vi "Main.vi"() -> ()   [LabVIEW 2020]
doc: "This template is for the Queued Message Handler design pattern.\n\nThe Event Handling Loop generates messages based on user interface actions.\n\nThe Message Handling Loop processes messages generated by the Event Handling Loop, or by other messages. The messages are string values, so new messages can be added easily to the Message Cases case structure in the Message Handling Loop. Each message cluster can also provide an optional value for Message Data, which is a variant that can be converted to whatever message-specific data is required."
uses:
  controls/Pressure Gauge.ctl
  controls/UI Data.ctl
  controls/UI State.ctl
  Settings/Settings.ctl
  controls/Hardware Configuration.ctl
  Logging/Logging Configuration.ctl
  <vilib>/Utility/error.llb/Error Cluster From Error Code.vi
  <vilib>/ErrorRing/Error Ring.xnode
  support/Message Queue/Message Queue.lvlib
  support/User Event - Stop/User Event - Stop.lvlib
  Acquisition/Acquisition.lvlib
  Control/Control.lvlib
  Logging/Logging.lvlib
  Settings/Settings.lvlib
panel:
  out "Valve State":bool[](array[boolean])
  out "T=":dbl format="%.2g"
  in  "Run Valve Sequence":bool
  out "P X-Ducer 7":dbl(knob) scale=0.0..5000.0 scale format="%.1p"
  out "P X-Ducer 6":dbl(knob) scale=0.0..5000.0 scale format="%.1p"
  out "P X-Ducer 5":dbl(knob) scale=0.0..5000.0 scale format="%.1p"
  out "P X-Ducer 4":dbl(knob) scale=0.0..5000.0 scale format="%.1p"
  out "P X-Ducer 3":dbl(knob) scale=0.0..5000.0 scale format="%.1p"
  out "P X-Ducer 2":dbl(knob) scale=0.0..5000.0 scale format="%.1p"
  out "P X-Ducer 1":dbl(knob) scale=0.0..5000.0 scale format="%.1p"
  out "P X-Ducer 0":T1 scale=0.0..5000.0 scale format="%.1p"
  in  "Settings":bool
  in  "Start":bool
  in  "Exit":bool
  # "River City Rocketry"
  # "Liquid Propulsion System Acquisition & Control"
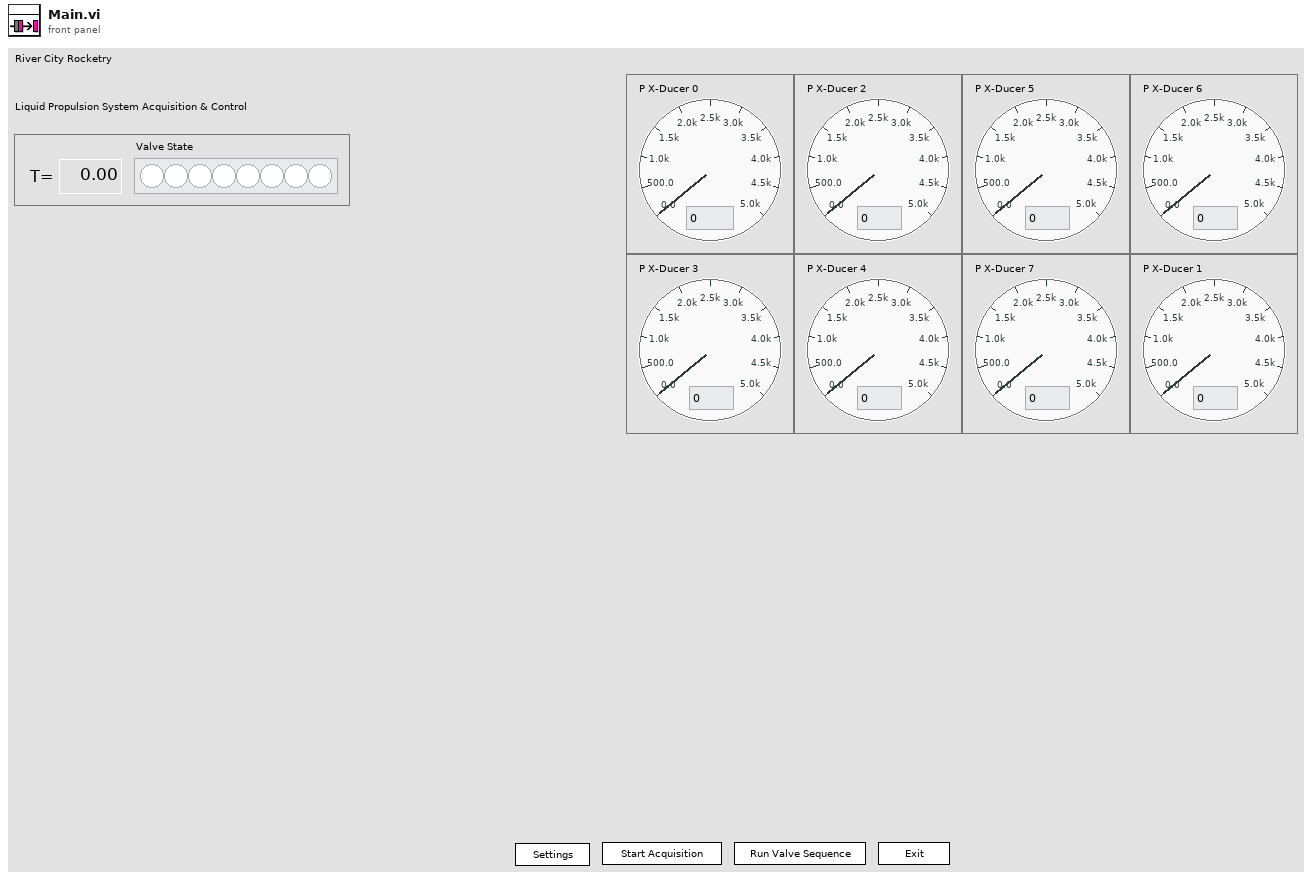
[diagram p1: front panel]
types:
  T1 = typedef "Pressure Gauge.ctl" = dbl
  T2 = typedef "Settings.lvlib/Settings.ctl" = cluster{"Hardware Configuration":T3, "Logging Configuration":T4}
  T3 = typedef "Acquisition.lvlib/Hardware Configuration.ctl" = cluster{"DAQmx Task":refnum<k21>, "Boolean":bool}
  T4 = typedef "Logging.lvlib/Logging Configuration.ctl" = cluster{"Log File Base Path":path, "TDMS File Reference":refnum<k34>, "Samples to Save":u32}
  T5 = typedef "UI State.ctl" = enum16{"Idle", "Acquiring and Logging", "Waiting for Exit", "Waiting for Exit (Acq Stopped)", "Waiting for Exit (Log Stopped)", "Waiting for Stop", "Waiting for Stop (Acq Stopped)", "Waiting for Stop (Log Stopped)"}
  T6 = typedef "UI Data.ctl" = cluster{"Settings Button Ref":refnum<vi>, "Start Button Ref":refnum<vi>, "Knob Refnum":refnum<vi>, "Knob Refnum 2":refnum<vi>, "Knob Refnum 3":refnum<vi>, "Knob Refnum 4":refnum<vi>, "Knob Refnum 5":refnum<vi>, "Knob Refnum 6":refnum<vi>, "Knob Refnum 7":refnum<vi>, "Knob Refnum 8":refnum<vi>, "Exit Button Refnum":refnum<vi>}
  T7 = typedef "Message Queue.lvlib/All Message Queues.ctl" = cluster{"Acquisition":refnum<queue>, "UI":refnum<queue>, "Control":refnum<queue>, "Logging":refnum<queue>}
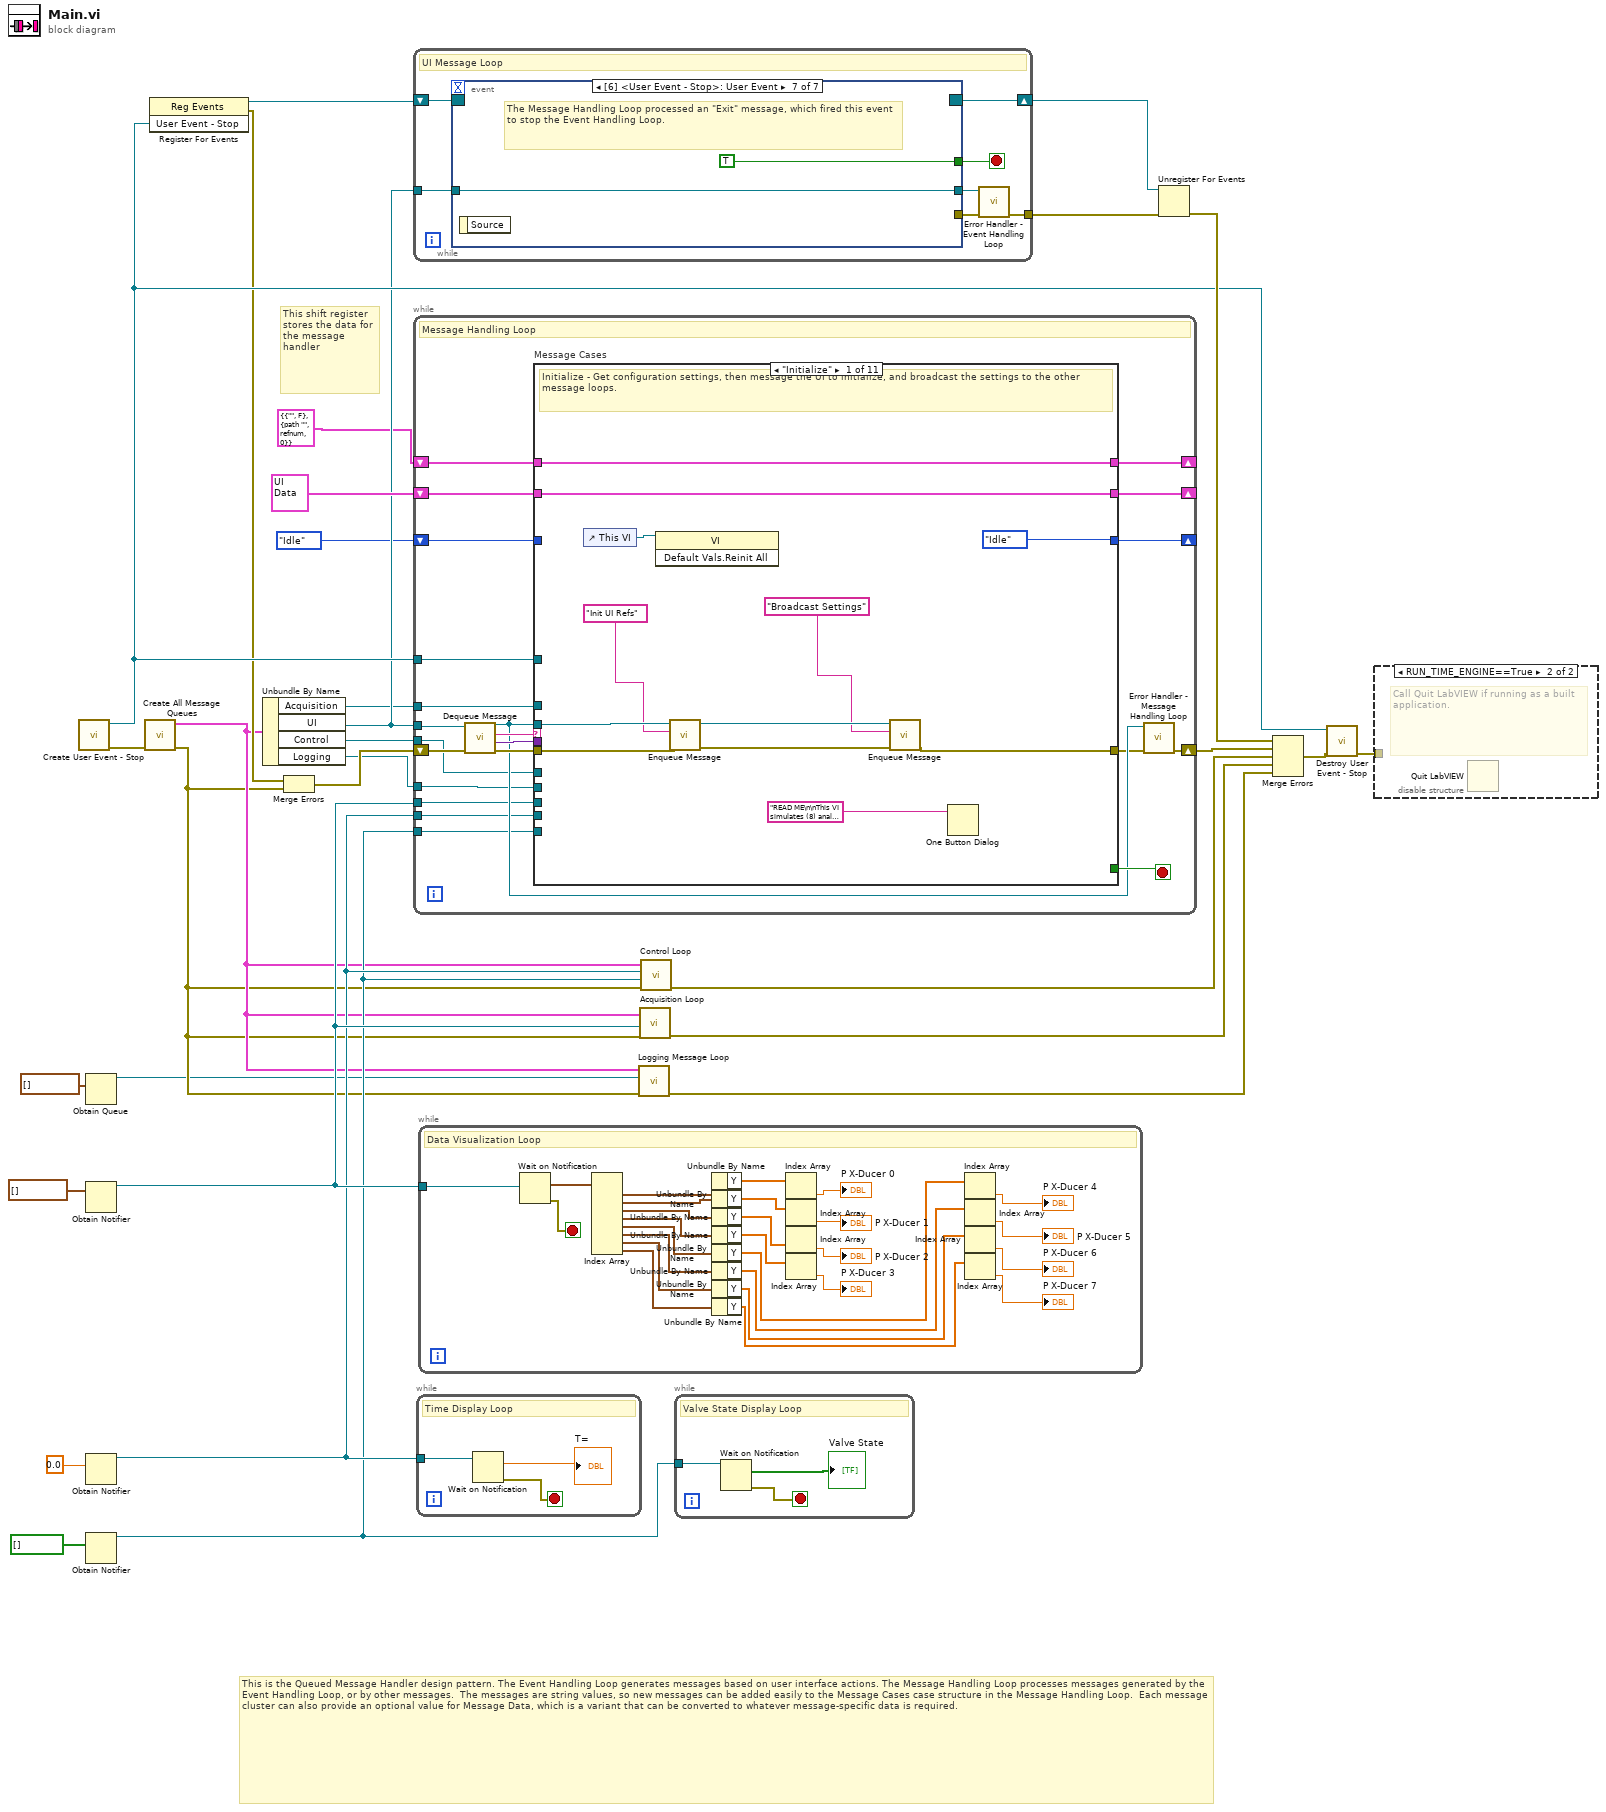
[diagram p0: block diagram]
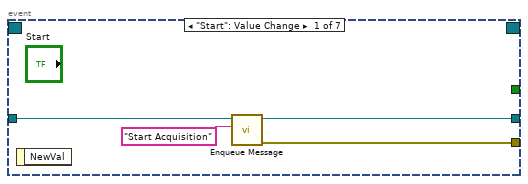
[diagram p3: hidden frame]
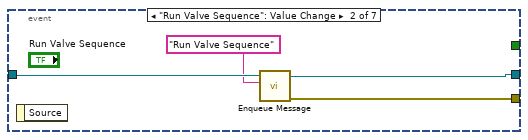
[diagram p4: hidden frame]
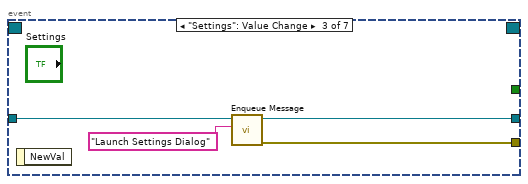
[diagram p5: hidden frame]
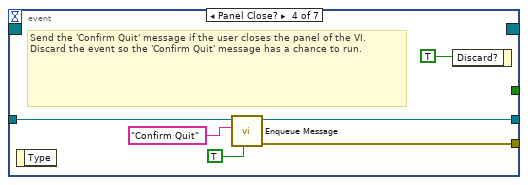
[diagram p6: hidden frame]
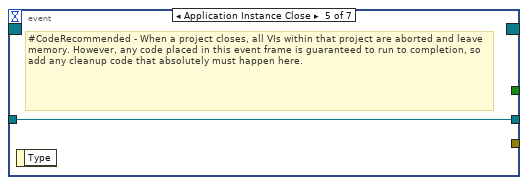
[diagram p7: hidden frame]
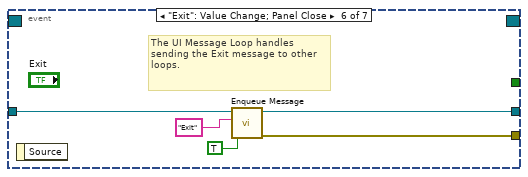
[diagram p8: hidden frame]
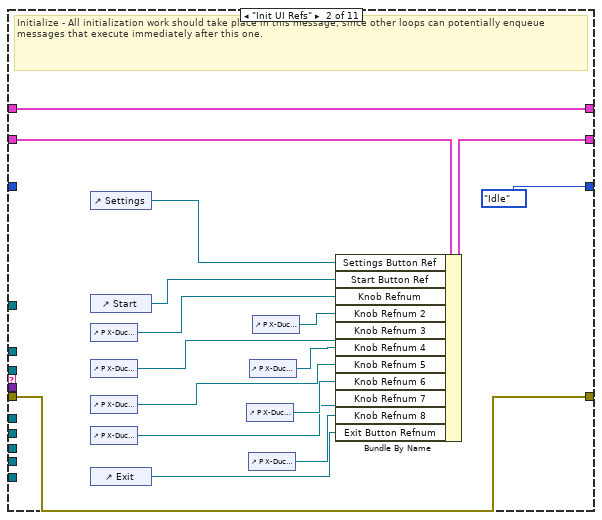
[diagram p9: hidden frame]
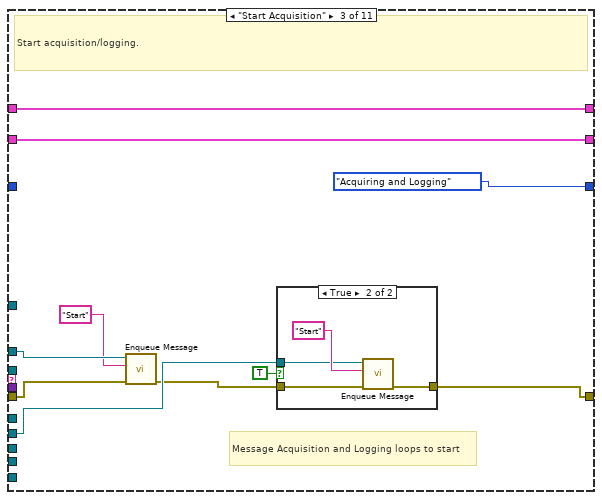
[diagram p10: hidden frame]
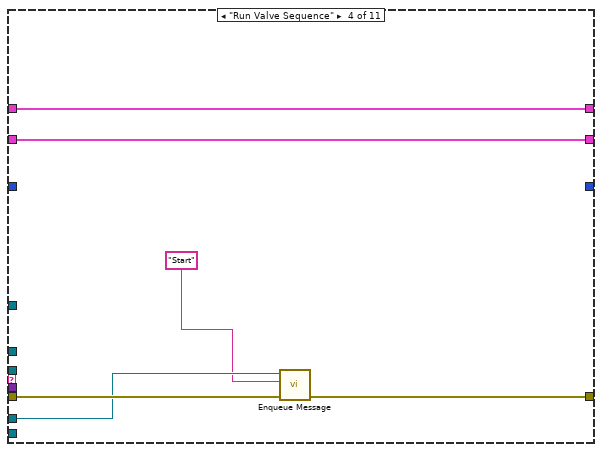
[diagram p12: hidden frame]
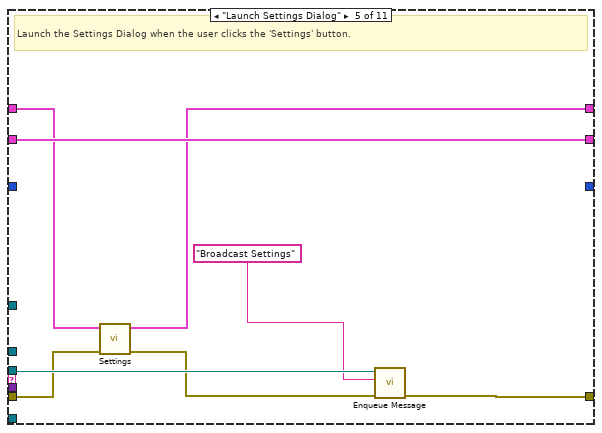
[diagram p13: hidden frame]
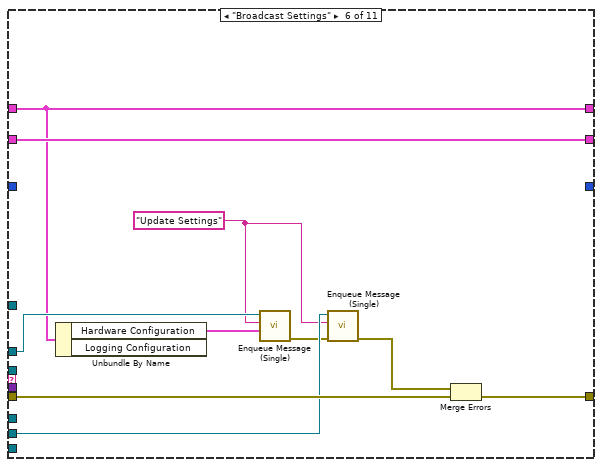
[diagram p14: hidden frame]
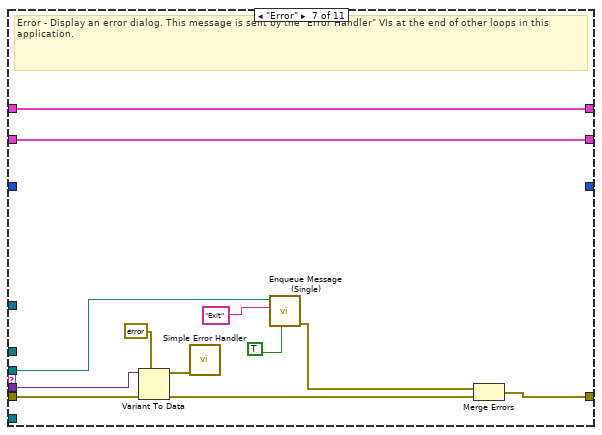
[diagram p15: hidden frame]
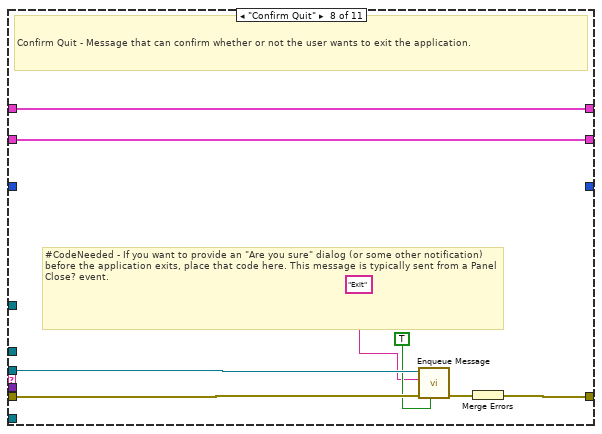
[diagram p16: hidden frame]
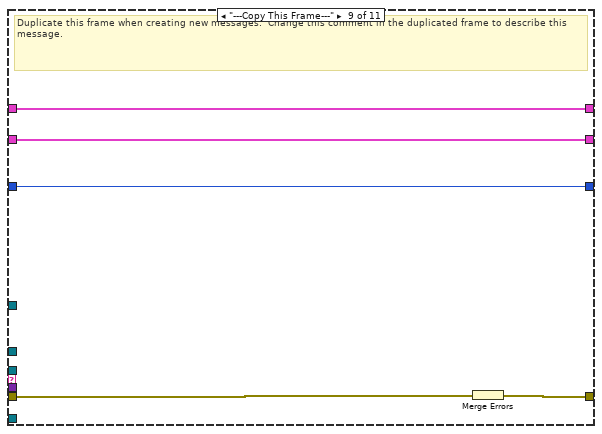
[diagram p17: hidden frame]
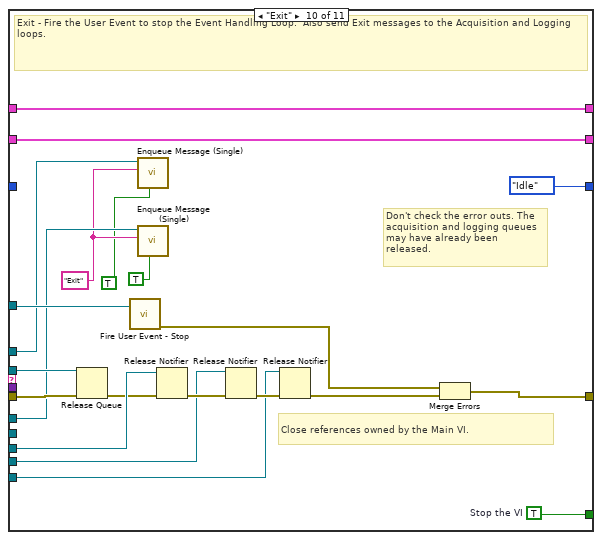
[diagram p18: hidden frame]
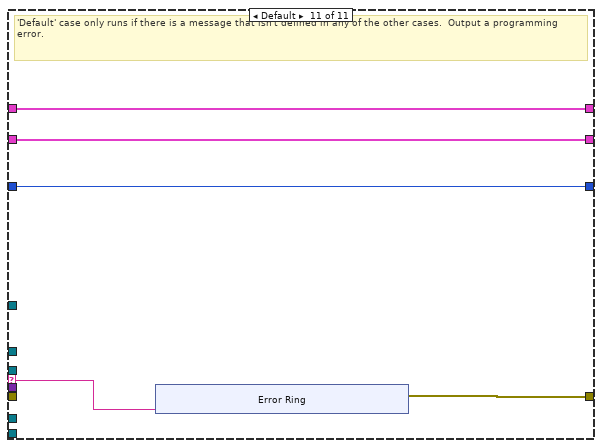
[diagram p19: hidden frame]
diagram:
  # "This is the Queued Message Handler design pattern. The Event Handling Loop generates messages based on user interface actions. The Message Handling Loop processes messages generated by the Event Handling Loop, or by other messages.  The messages are string values, so new messages can be added easily to the Message Cases case structure in the Message Handling Loop.  Each message cluster can also provide an optional value for Message Data, which is a variant that can be converted to whatever message-specific data is required."
  # "This shift register stores the data for the message handler"
  n1 = call "Create User Event - Stop.vi"() -> ("error out"=w18:errorcluster, "User Event - Stop"=w23:refnum<user-event>)  [unwired: 10 in]
  n2 = Obtain Queue(element data type=waveform(dbl)[] []) -> (queue out=w2:refnum<queue>)  [unwired: 4 in, 2 out]
  n3 = Obtain Notifier(notification data type=waveform(dbl)[] []) -> (notifier out=w11:refnum<notifier>)  [unwired: 3 in, 2 out]
  n4 = Obtain Notifier(notification data type=0.0) -> (notifier out=w9:refnum<notifier>)  [unwired: 3 in, 2 out]
  n5 = Obtain Notifier(notification data type=bool[] [] ("Array")) -> (notifier out=w8:refnum<notifier>)  [unwired: 3 in, 2 out]
  n6 = call "Create All Message Queues.vi"("error in (no error)"=w18) -> ("error out"=w5:errorcluster, "Message Queues out"=w6:T7)  [unwired: 9 in]
  n7 = register-events(w23) -> (reference out=w24:refnum<event-registration>, error out=w21:errorcluster)  [unwired: 2 in]
  n8 = Unbundle By Name(w6) -> ("Acquisition"=w17:refnum<queue>, "UI"=w20:refnum<queue>, "Control"=w13:refnum<queue>, "Logging"=w7:refnum<queue>)
  n9 = Merge Errors(w21, w5) -> (w22:errorcluster)
  n10 = while {
    tunnel: w20 -> [w38]
    shift-right: [w36] -> w28
    shift-left: w24 -> [w37]
    tunnel: [w32] -> w25
    stop <- w34 stop-if-true
    # "UI Message Loop"
    n11 = event shown="[6] <User Event - Stop>: User Event" {
      selector: w37 -> [_ _ _ _ _ _ _]
      dyn-events: [_ _ _ _ _ _ _] -> w36
      timeout: _ -> [_ _ _ _ _ _ _]
      tunnel: [_ _ _ _ _ _ TRUE ("Discard?")] -> w34
      tunnel: w38 -> [w42 w46 w50 w55 w57 w62 w64]
      tunnel: [w39 w44 w47 w54 _ w61 _] -> w35
      tunnel: [w41 w45 w49 w53 w57 w60 w64] -> w33
      event "Start": Value Change {
        n12 = event-data() -> ()  [unwired: 1 in, 1 out]
        n13 = call-poly "Enqueue Message.vi"("Message"="Start Acquisition", "Message Queue"=w42) -> ("error out"=w39:errorcluster, "dup Message Queue"=w41:refnum<queue>)  [unwired: 8 in]
      }
      event "Run Valve Sequence": Value Change {
        n14 = event-data() -> ()  [unwired: 1 in, 1 out]
        n15 = call-poly "Enqueue Message.vi"("Message"="Run Valve Sequence", "Message Queue"=w46) -> ("error out"=w44:errorcluster, "dup Message Queue"=w45:refnum<queue>)  [unwired: 8 in]
      }
      event "Settings": Value Change {
        n16 = event-data() -> ()  [unwired: 1 in, 1 out]
        n17 = call-poly "Enqueue Message.vi"("Message"="Launch Settings Dialog", "Message Queue"=w50) -> ("error out"=w47:errorcluster, "dup Message Queue"=w49:refnum<queue>)  [unwired: 8 in]
      }
      event Panel Close? {
        # "Send the 'Confirm Quit' message if the user closes the panel of the VI. Discard the event so the 'Confirm Quit' message has a chance to run."
        n18 = event-data() -> ()  [unwired: 1 in, 1 out]
        n19 = call-poly "Enqueue Message.vi"("Priority Message? (F)"=TRUE, "Message"="Confirm Quit", "Message Queue"=w55) -> ("error out"=w54:errorcluster, "dup Message Queue"=w53:refnum<queue>)  [unwired: 7 in]
        n20 = event-data("Discard?"=TRUE) -> ()  [unwired: 1 in, 1 out]
      }
      event Application Instance Close {
        # "#CodeRecommended - When a project closes, all VIs within that project are aborted and leave memory. However, any code placed in this event frame is guaranteed to run to completion, so add any cleanup code that absolutely must happen here."
        n21 = event-data() -> ()  [unwired: 1 in, 1 out]
      }
      event "Exit": Value Change; Panel Close {
        # "The UI Message Loop handles sending the Exit message to other loops."
        n22 = event-data() -> ()  [unwired: 1 in, 1 out]
        n23 = call-poly "Enqueue Message.vi"("Priority Message? (F)"=TRUE, "Message"="Exit", "Message Queue"=w62) -> ("error out"=w61:errorcluster, "dup Message Queue"=w60:refnum<queue>)  [unwired: 7 in]
      }
      event User Event {
        # "The Message Handling Loop processed an \"Exit\" message, which fired this event to stop the Event Handling Loop."
        n24 = event-data() -> ()  [unwired: 1 in, 1 out]
      }
    }
    n25 = call "Error Handler - Event Handling Loop.vi"("error in (no error)"=w35, "Message Queue"=w33) -> ("dup error in"=w32:errorcluster)  [unwired: 8 in, 1 out]
  }
  n26 = while {
    tunnel: w20 -> [w78]
    shift-right: [w85] -> _
    shift-left: T6 {"Settings Button Ref"=refnum, "Start Button Ref"=refnum, "Knob Refnum"=refnum, "Knob Refnum 2"=refnum, "Knob Refnum 3"=refnum, "Knob Refnum 4"=refnum, "Knob Refnum 5"=refnum, "Knob Refnum 6"=refnum, "Knob Refnum 7"=refnum, "Knob Refnum 8"=refnum, "Exit Button Refnum"=refnum} ("Data Cluster") -> [w86]
    tunnel: w23 -> [w83]
    tunnel: w17 -> [w74]
    shift-right: [w72] -> _
    shift-left: T2 {"Hardware Configuration"={"DAQmx Task"="", "Boolean"=FALSE}, "Logging Configuration"={"Log File Base Path"=path "", "TDMS File Reference"=refnum, "Samples to Save"=0}} ("Settings") -> [w73]
    shift-right: [w76] -> w31
    shift-left: w22 -> [w82]
    tunnel: w11 -> [w71]
    shift-right: [w69] -> _
    shift-left: UI_State."Idle" ("UI State") -> [w70]
    tunnel: w13 -> [w68]
    tunnel: w9 -> [w67]
    tunnel: w8 -> [w66]
    tunnel: w7 -> [w65]
    stop <- w84 stop-if-true
    # "Message Handling Loop"
    n27 = call "Dequeue Message.vi"("error in (no error)"=w82, "Message Queue"=w78) -> ("error out"=w81:errorcluster, "Message Data"=w79:variant, "Message"=w80:string, "dup Message Queue"=w77:refnum<queue>)  [unwired: 6 in]
    n28 = case "Message Cases" shown="\"Initialize\"" w80 {
      selector: w80 -> [_ _ _ _ _ _ _ _ _ _ w202]
      tunnel: w77 -> [w97 _ _ _ w142 _ w157 w169 _ w199 _]
      tunnel: w81 -> [w95 w111 w123 w133 w138 w151 w165 w173 w178 w193 _]
      tunnel: [w93 w111 w116 w132 w139 w150 w159 w171 w176 w196 w203] -> w75
      tunnel: w86 -> [w98 w114 w124 w135 w143 w153 w164 w172 w177 w198 w204]
      tunnel: [w98 w113 w124 w135 w143 w153 w164 w172 w177 w198 w204] -> w85
      tunnel: [_ _ _ _ _ _ _ _ _ w197 _] -> w84
      tunnel: w79 -> [_ _ _ _ _ _ w163 _ _ _ _]
      tunnel: w83 -> [_ _ _ _ _ _ _ _ _ w195 _]
      tunnel: w74 -> [_ _ w121 _ _ w152 _ _ _ w192 _]
      tunnel: [w90 w112 w122 w134 w140 w149 w158 w166 w175 w191 w201] -> w72
      tunnel: w73 -> [w90 w112 w122 w134 w136 w149 w158 w166 w175 w191 w201]
      tunnel: w71 -> [_ _ _ _ _ _ _ _ _ w190 _]
      tunnel: w70 -> [_ _ _ _ _ _ _ _ w174 _ w200]
      tunnel: [UI_State."Idle" ("UI State") UI_State."Idle" ("UI State") UI_State."Acquiring and Logging" ("UI State") _ _ _ _ _ w174 UI_State."Idle" ("UI State") w200] -> w69
      tunnel: w68 -> [_ _ _ w131 _ _ _ _ _ w187 _]
      tunnel: w67 -> [_ _ _ _ _ _ _ _ _ w181 _]
      tunnel: w66 -> [_ _ _ _ _ _ _ _ _ w180 _]
      tunnel: w65 -> [_ _ w118 _ _ w148 _ _ _ _ _]
      frame "Initialize" {
        # "Initialize - Get configuration settings, then message the UI to initialize, and broadcast the settings to the other message loops."
        n29 = control-ref of="This VI"() -> (w88:refnum<vi>)
        n30 = invoke class="VI" method="Default Vals.Reinit All"(reference=w88) -> ()  [unwired: 2 in, 3 out]
        n31 = call-poly "Enqueue Message.vi"("error in (no error)"=w95, "Message"="Init UI Refs", "Message Queue"=w97) -> ("error out"=w94:errorcluster, "dup Message Queue"=w96:refnum<queue>)  [unwired: 7 in]
        n32 = call-poly "Enqueue Message.vi"("error in (no error)"=w94, "Message"="Broadcast Settings", "Message Queue"=w96) -> ("error out"=w93:errorcluster)  [unwired: 7 in, 1 out]
        n33 = One Button Dialog(message="READ ME\n\nThis VI simulates (8) analog input channels and (8) digital output channels. When 'Run Valve Sequence' is pressed, a pre-programmed digital output sequence starts. The sequence is hard-coded into the Digital Ouput sub-VI. \nTasks are configured in the Measurement & Automation Explorer (NI MAX). \n\nUpcoming:\n-Proper settings menu that allows task selection for each channel type, setting the countdown, and settings for logging data to file\n-Fixed exit/stop button\n-Allow users to edit valve sequence\n-File logging\n") -> ()  [unwired: 1 in, 1 out]
      }
      frame "Init UI Refs" {
        # "Initialize - All initialization work should take place in this message, since other loops can potentially enqueue messages that execute immediately after this one."
        n34 = control-ref of="Settings"() -> (w109:refnum<vi>)
        n35 = control-ref of="Start"() -> (w108:refnum<vi>)
        n36 = control-ref of="P X-Ducer 0"() -> (w107:refnum<vi>)
        n37 = control-ref of="P X-Ducer 2"() -> (w105:refnum<vi>)
        n38 = control-ref of="P X-Ducer 4"() -> (w103:refnum<vi>)
        n39 = control-ref of="P X-Ducer 6"() -> (w101:refnum<vi>)
        n40 = control-ref of="Exit"() -> (w99:refnum<vi>)
        n41 = control-ref of="P X-Ducer 5"() -> (w102:refnum<vi>)
        n42 = control-ref of="P X-Ducer 7"() -> (w100:refnum<vi>)
        n43 = control-ref of="P X-Ducer 3"() -> (w104:refnum<vi>)
        n44 = control-ref of="P X-Ducer 1"() -> (w106:refnum<vi>)
        n45 = Bundle By Name(cluster=w114, "Settings Button Ref"=w109, "Start Button Ref"=w108, "Knob Refnum"=w107, "Knob Refnum 2"=w106, "Knob Refnum 3"=w105, "Knob Refnum 4"=w104, "Knob Refnum 5"=w103, "Knob Refnum 6"=w102, "Knob Refnum 7"=w101, "Knob Refnum 8"=w100, "Exit Button Refnum"=w99) -> (w113:T6)
      }
      frame "Start Acquisition" {
        # "Message Acquisition and Logging loops to start"
        # "Start acquisition/logging."
        n46 = call-poly "Enqueue Message.vi"("error in (no error)"=w123, "Message"="Start" ("\"Do Something\" button pressed"), "Message Queue"=w121) -> ("error out"=w117:errorcluster)  [unwired: 7 in, 1 out]
        n47 = case shown="True" TRUE {
          tunnel: w118 -> [_ w128]
          tunnel: w117 -> [w125 w127]
          tunnel: [w125 w126] -> w116
          frame False {
          }
          frame True {
            n48 = call-poly "Enqueue Message.vi"("error in (no error)"=w127, "Message"="Start" ("\"Do Something\" button pressed"), "Message Queue"=w128) -> ("error out"=w126:errorcluster)  [unwired: 7 in, 1 out]
          }
        }
      }
      frame "Run Valve Sequence" {
        n49 = call-poly "Enqueue Message.vi"("error in (no error)"=w133, "Message"="Start", "Message Queue"=w131) -> ("error out"=w132:errorcluster)  [unwired: 7 in, 1 out]
      }
      frame "Launch Settings Dialog" {
        # "Launch the Settings Dialog when the user clicks the 'Settings' button."
        n50 = call "Settings.vi"("error in (no error)"=w138, "Settings In"=w136) -> ("error out"=w137:errorcluster, "Settings Out"=w140:T2)  [unwired: 8 in]
        n51 = call-poly "Enqueue Message.vi"("error in (no error)"=w137, "Message"="Broadcast Settings", "Message Queue"=w142) -> ("error out"=w139:errorcluster)  [unwired: 7 in, 1 out]
      }
      frame "Broadcast Settings" {
        w144 = "Update Settings"
        n52 = Unbundle By Name(w149) -> ("Hardware Configuration"=w145:T3)  [unwired: 1 out]
        n53 = call "Enqueue Message (Single).vi"("Message Data"=w145, "Message"=w144, "Message Queue"=w152) -> ("error out"=w147:errorcluster)  [unwired: 7 in, 1 out]
        n54 = call "Enqueue Message (Single).vi"("error in (no error)"=w147, "Message"=w144, "Message Queue"=w148) -> ("error out"=w146:errorcluster)  [unwired: 7 in, 1 out]
        n55 = Merge Errors(w146, w151) -> (w150:errorcluster)
      }
      frame "Error" {
        # "Error - Display an error dialog. This message is sent by the \"Error Handler\" VIs at the end of other loops in this application."
        n56 = Variant To Data(error in=w165, type=errorcluster {"status"=FALSE, "code"=0, "source"=""} ("error constant"), Variant=w163) -> (data=w161:errorcluster, error out=w160:errorcluster)
        n57 = call <vilib>:"Simple Error Handler.vi"("error in (no error)"=w161) -> ()  [unwired: 4 in, 5 out]
        n58 = call "Enqueue Message (Single).vi"("Priority Message? (F)"=TRUE, "Message"="Exit", "Message Queue"=w157) -> ("error out"=w154:errorcluster)  [unwired: 7 in, 1 out]
        n59 = Merge Errors(w154, w160) -> (w159:errorcluster)
      }
      frame "Confirm Quit" {
        # "#CodeNeeded - If you want to provide an \"Are you sure\" dialog (or some other notification) before the application exits, place that code here. This message is typically sent from a Panel Close? event."
        # "Confirm Quit - Message that can confirm whether or not the user wants to exit the application."
        n60 = call-poly "Enqueue Message.vi"("Priority Message? (F)"=TRUE, "error in (no error)"=w173, "Message"="Exit", "Message Queue"=w169) -> ("error out"=w170:errorcluster)  [unwired: 6 in, 1 out]
        n61 = Merge Errors(w170) -> (w171:errorcluster)
      }
      frame "---Copy This Frame---" {
        # "Duplicate this frame when creating new messages.  Change this comment in the duplicated frame to describe this message."
        n62 = Merge Errors(w178) -> (w176:errorcluster)
      }
      frame "Exit" {
        w186 = "Exit"
        w197 = TRUE  # Stop the VI
        # "Don't check the error outs. The acquisition and logging queues may have already been released."
        # "Close references owned by the Main VI."
        # "Exit - Fire the User Event to stop the Event Handling Loop.  Also send Exit messages to the Acquisition and Logging loops."
        n63 = Release Queue(queue=w199, error in (no error)=w193) -> (error out=w189:errorcluster)  [unwired: 1 in, 2 out]
        n64 = call "Fire User Event - Stop.vi"("User Event - Stop"=w195) -> ("error out"=w194:errorcluster)  [unwired: 10 in]
        n65 = call "Enqueue Message (Single).vi"("Priority Message? (F)"=TRUE, "Message"=w186, "Message Queue"=w192) -> ()  [unwired: 7 in, 2 out]
        n66 = call "Enqueue Message (Single).vi"("Priority Message? (F)"=TRUE, "Message"=w186, "Message Queue"=w187) -> ()  [unwired: 7 in, 2 out]
        n67 = Release Notifier(notifier=w190, error in (no error)=w189) -> (error out=w184:errorcluster)  [unwired: 1 in, 2 out]
        n68 = Release Notifier(notifier=w181, error in (no error)=w184) -> (error out=w183:errorcluster)  [unwired: 1 in, 2 out]
        n69 = Release Notifier(notifier=w180, error in (no error)=w183) -> (error out=w182:errorcluster)  [unwired: 1 in, 2 out]
        n70 = Merge Errors(w194, w182) -> (w196:errorcluster)
      }
      frame Default {
        # "'Default' case only runs if there is a message that isn't defined in any of the other cases.  Output a programming error."
        n71 = xnode "Error Ring"("parameter 0"=w202) -> ("error out"=w203:errorcluster)
      }
    }
    n72 = call "Error Handler - Message Handling Loop.vi"("error in (no error)"=w75, "Message Queue"=w77) -> ("dup error in"=w76:errorcluster)  [unwired: 8 in, 1 out]
  }
  n73 = while {
    tunnel: w9 -> [w213]
    stop <- w212 stop-if-true
    # "Time Display Loop"
    n74 = Wait on Notification(notifier=w213) -> (notification=→"T=":dbl, error out=w212:errorcluster)  [unwired: 3 in, 2 out]
  }
  n75 = while {
    tunnel: w11 -> [w215]
    stop <- w216 stop-if-true
    # "Data Visualization Loop"
    n76 = Wait on Notification(notifier=w215) -> (notification=w241:waveform(dbl)[], error out=w216:errorcluster)  [unwired: 3 in, 2 out]
    n77 = Index Array(array=w241) -> (element #1=w240:waveform(dbl), element #2=w238:waveform(dbl), element #3=w235:waveform(dbl), element #4=w234:waveform(dbl), element #5=w233:waveform(dbl), element #6=w232:waveform(dbl), element #7=w231:waveform(dbl), element #8=w230:waveform(dbl))  [unwired: 8 in]
    n78 = Unbundle By Name(w240) -> ("Y"=w239:dbl[])
    n79 = Unbundle By Name(w238) -> ("Y"=w237:dbl[])
    n80 = Unbundle By Name(w235) -> ("Y"=w236:dbl[])
    n81 = Unbundle By Name(w234) -> ("Y"=w229:dbl[])
    n82 = Unbundle By Name(w233) -> ("Y"=w228:dbl[])
    n83 = Unbundle By Name(w232) -> ("Y"=w227:dbl[])
    n84 = Unbundle By Name(w231) -> ("Y"=w226:dbl[])
    n85 = Unbundle By Name(w230) -> ("Y"=w225:dbl[])
    n86 = Index Array(array=w239) -> (element=→"P X-Ducer 0":dbl)  [unwired: 1 in]
    n87 = Index Array(array=w237) -> (element=→"P X-Ducer 1":dbl)  [unwired: 1 in]
    n88 = Index Array(array=w236) -> (element=→"P X-Ducer 2":dbl)  [unwired: 1 in]
    n89 = Index Array(array=w229) -> (element=→"P X-Ducer 3":dbl)  [unwired: 1 in]
    n90 = Index Array(array=w228) -> (element=→"P X-Ducer 4":dbl)  [unwired: 1 in]
    n91 = Index Array(array=w227) -> (element=→"P X-Ducer 5":dbl)  [unwired: 1 in]
    n92 = Index Array(array=w226) -> (element=→"P X-Ducer 6":dbl)  [unwired: 1 in]
    n93 = Index Array(array=w225) -> (element=→"P X-Ducer 7":dbl)  [unwired: 1 in]
  }
  n94 = call "Logging Message Loop.vi"("error in (no error)"=w5, "Data Queue"=w2, "Message Queues"=w6) -> ("error out"=w4:errorcluster)  [unwired: 8 in]
  n95 = call "Acquisition Loop.vi"("error in (no error)"=w5, "Data Notifier"=w11, "Message Queues"=w6) -> ("error out"=w14:errorcluster)  [unwired: 8 in]
  n96 = call "Control Loop.vi"("error in (no error)"=w5, "valve state notifier"=w8, "notifier"=w9, "Message Queues"=w6) -> ("error out"=w15:errorcluster)  [unwired: 7 in]
  n97 = while {
    tunnel: w8 -> [w244]
    stop <- w242 stop-if-true
    # "Valve State Display Loop"
    n98 = Wait on Notification(notifier=w244) -> (notification=→"Valve State":bool[], error out=w242:errorcluster)  [unwired: 3 in, 2 out]
  }
  n99 = Unregister For Events(event registration refnum=w28, error in=w25) -> (error out=w29:errorcluster)
  n100 = Merge Errors(w29, w31, w15, w14, w4) -> (w30:errorcluster)
  n101 = call "Destroy User Event - Stop.vi"("error in (no error)"=w30, "User Event - Stop"=w23) -> ("error out"=w26:errorcluster)  [unwired: 9 in]
  n102 = disable-structure shown="RUN_TIME_ENGINE==True" {
    disable-tunnel: w26 -> [_ _]
    frame condition #0 (active) {
    }
    frame condition #1 {
      # "Call Quit LabVIEW if running as a built application."
      n103 = Quit LabVIEW() -> ()  [unwired: 1 in]
    }
  }
